vi "Read LSEConfig.vi"(8 "error in (no error)":errorcluster, 11 "LSEPlugin in":refnum<class "LSEPlugin.lvclass">) -> (0 "error out":errorcluster, 2 "LSEConfig":T1={"NoiseVariance"=0.0, "IEEESystem"=39, "PMULocations"=[16], "Vindex"=0, "Iindex"=3, "DynamicRef"=""}, 3 "LSEPlugin out":refnum<class "LSEPlugin.lvclass">)   [LabVIEW 2017, in "AppPlugins.lvlib" / "LSEPlugin.lvclass"]
uses:
  LSEPlugin.lvclass
  PublicAPI/Typedefs/LSEConfig.ctl
  LSEPlugin.lvclass/LSEPlugin.ctl
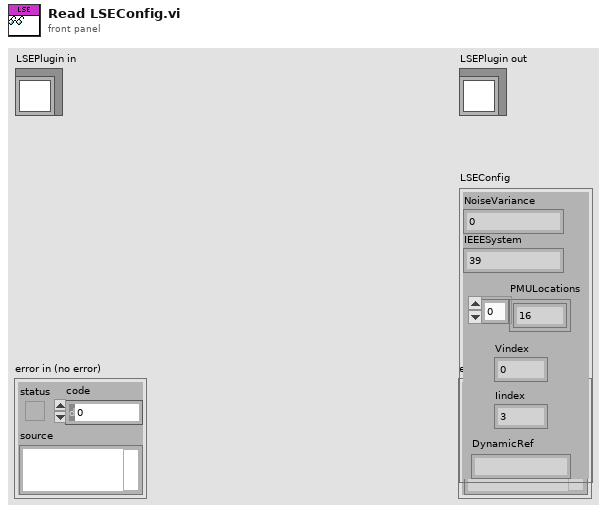
[diagram p1: front panel]
types:
  T1 = typedef "AppPlugins.lvlib/LSEPlugin.lvclass/LSEConfig.ctl" = cluster{"NoiseVariance":dbl, "IEEESystem":u32, "PMULocations":u32[], "Vindex":i32, "Iindex":i32, "DynamicRef":string}
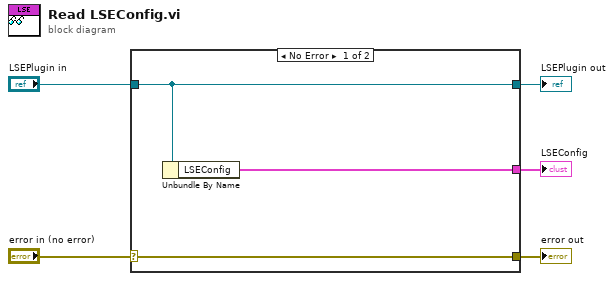
[diagram p0: block diagram]
diagram:
  n1 = case shown="No Error" "error in (no error)" {
    selector: "error in (no error)" -> [w8 w9]
    tunnel: [w8 w9] -> w4
    tunnel: [w7 w10] -> w2
    tunnel: "LSEPlugin in" -> [w7 w10]
    tunnel: [w6 _] -> w1
    frame No Error {
      n2 = Unbundle By Name(w7) -> ("LSEConfig"=w6:T1)
    }
    frame Error {
    }
  }
  "error out" <- w4
  "LSEPlugin out" <- w2
  "LSEConfig" <- w1
